vi "Baseline Thresholding.vi"(4 "Baseline Threshold Parameters":T1={"Current"=[20, 20, 20, 20, 20], "Pulse Duration"=[500, 500, 500, 500]}, 5 "Stimulator":T5={"Stim Open Data"={"Name"="", "Mode"=enum."LIVE", "Visa Timeout"=0}, "Stim Init Data"={"Frequency"=0.0, "N Factor"=0, "D/T Int"=0.0, "Active Channels"=[], "LF Channels"=[]}, "Stim Update Data"={"Pulse Mode"=[enum."Single"], "Current"=[], "Pulse Dur"=[]}, "Stim Status"={"Open"=FALSE, "On"=FALSE}}) -> (1 "Baseline Threshold Params Out":T1={"Current"=[20, 20, 20, 20, 20], "Pulse Duration"=[500, 500, 500, 500]} caption="Final Parameters", 2 "Stimulator Out":T5={"Stim Open Data"={"Name"="", "Mode"=enum."LIVE", "Visa Timeout"=0}, "Stim Init Data"={"Frequency"=0.0, "N Factor"=0, "D/T Int"=0.0, "Active Channels"=[], "LF Channels"=[]}, "Stim Update Data"={"Pulse Mode"=[enum."Single"], "Current"=[], "Pulse Dur"=[]}, "Stim Status"={"Open"=FALSE, "On"=FALSE}})   [LabVIEW 2019]
uses:
  Version 2/Data Type Defs/Stimulator.ctl
  Version 2/Data Type Defs/Stim Open Data.ctl
  Version 2/Data Type Defs/Stim Init Data.ctl
  Version 2/Data Type Defs/Stim Update Data.ctl
  Version 2/Data Type Defs/Pulse Mode (array).ctl
  Version 2/Data Type Defs/Stim Status.ctl
  Controls/Type Defs/Baseline Threshold Params.ctl
  Controls/Stim Current Array.ctl
  Controls/Pulse Duration Array.ctl
panel:
  out "Stim Open Data.Mode":enum16{"LIVE", "SIM"}(ring)
  out "Stimulator":refnum<visa-resource-name>
  out "Final Parameters":T1={"Current"=[20, 20, 20, 20, 20], "Pulse Duration"=[500, 500, 500, 500]}
  in  "Controls":T4={"Channel"=[], "PW"=340, "Current"=60} {"Current" max=126 step=2; "PW" min=20 max=500 step=5 scale=0.0..500.0}
  in  "Done":bool
  # "Gluteals"
  # "Hamstrings"
  # "Quads"
  # "TA/Dorsi"
  # "TS/Plantar"
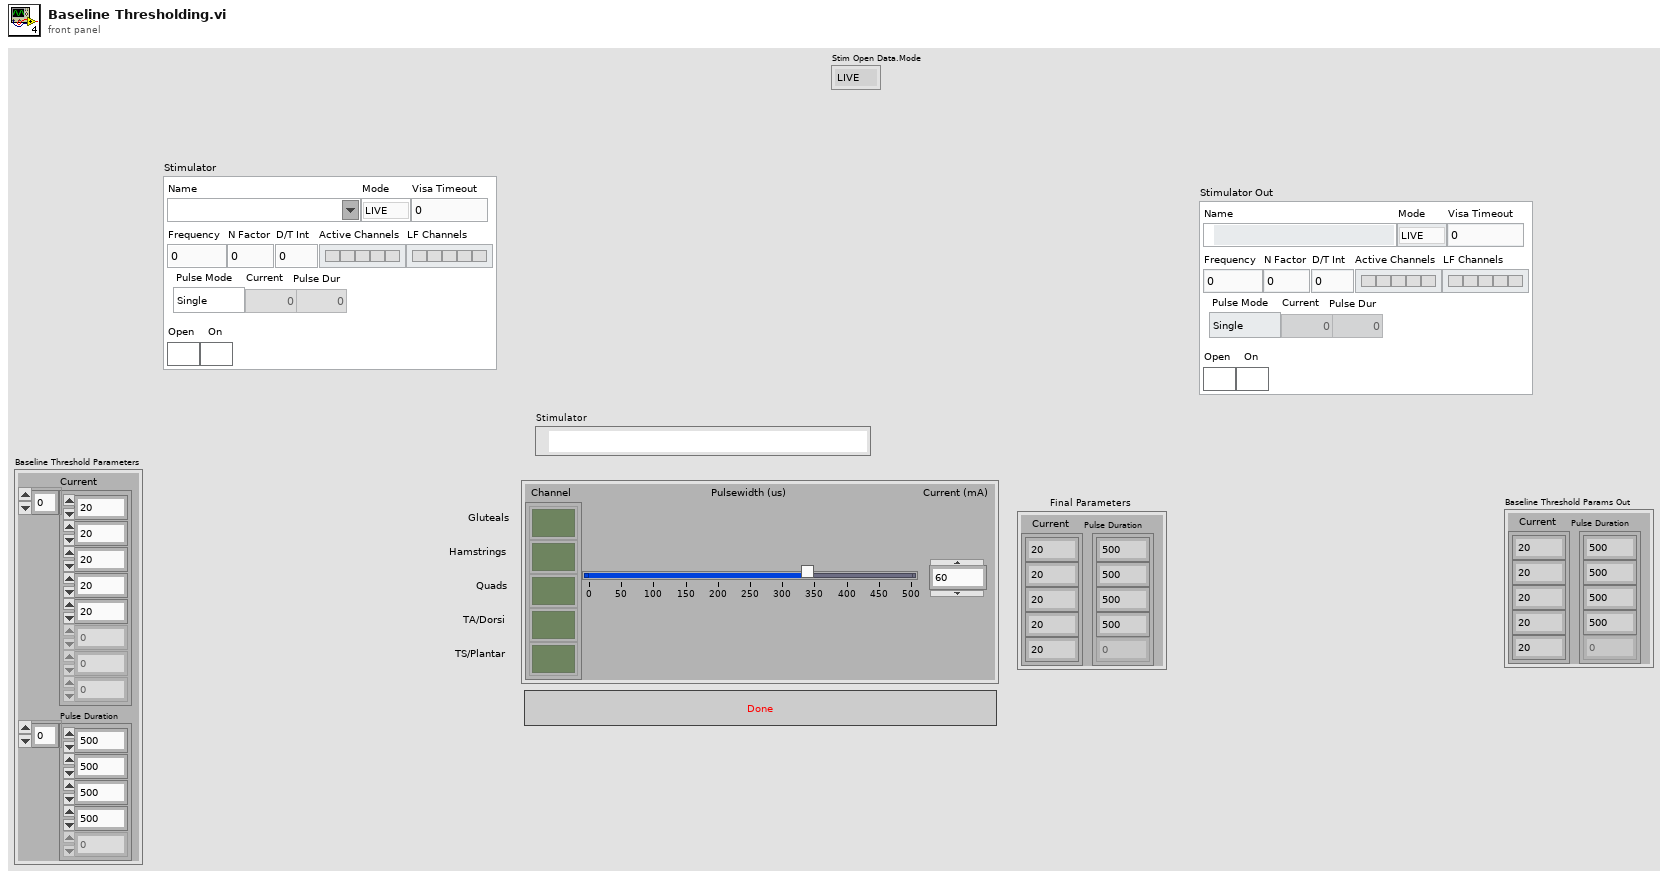
[diagram p1: front panel]
types:
  T1 = typedef "Baseline Threshold Params.ctl" = cluster{"Current":T2, "Pulse Duration":T3}
  T2 = typedef "Stim Current Array.ctl" = u8[]
  T3 = typedef "Pulse Duration Array.ctl" = u32[]
  T4 = cluster{"Channel":bool[], "PW":u16, "Current":u8}
  T5 = typedef "Stimulator.ctl" = cluster{"Stim Open Data":T6, "Stim Init Data":T7, "Stim Update Data":T8, "Stim Status":T10}
  T6 = typedef "Stim Open Data.ctl" = cluster{"Name":refnum<visa-resource-name>, "Mode":enum16{"LIVE", "SIM"}, "Visa Timeout":u32}
  T7 = typedef "Stim Init Data.ctl" = cluster{"Frequency":dbl, "N Factor":u8, "D/T Int":dbl, "Active Channels":bool[], "LF Channels":bool[]}
  T8 = typedef "Stim Update Data.ctl" = cluster{"Pulse Mode":T9, "Current":u32[], "Pulse Dur":u32[]}
  T9 = typedef "Pulse Mode (array).ctl" = enum16{"Single", "Doublet", "Triplet"}[]
  T10 = typedef "Stim Status.ctl" = cluster{"Open":bool, "On":bool}
  T11 = enum8{"Enabled", "Disabled", "Disabled and Grayed Out"}
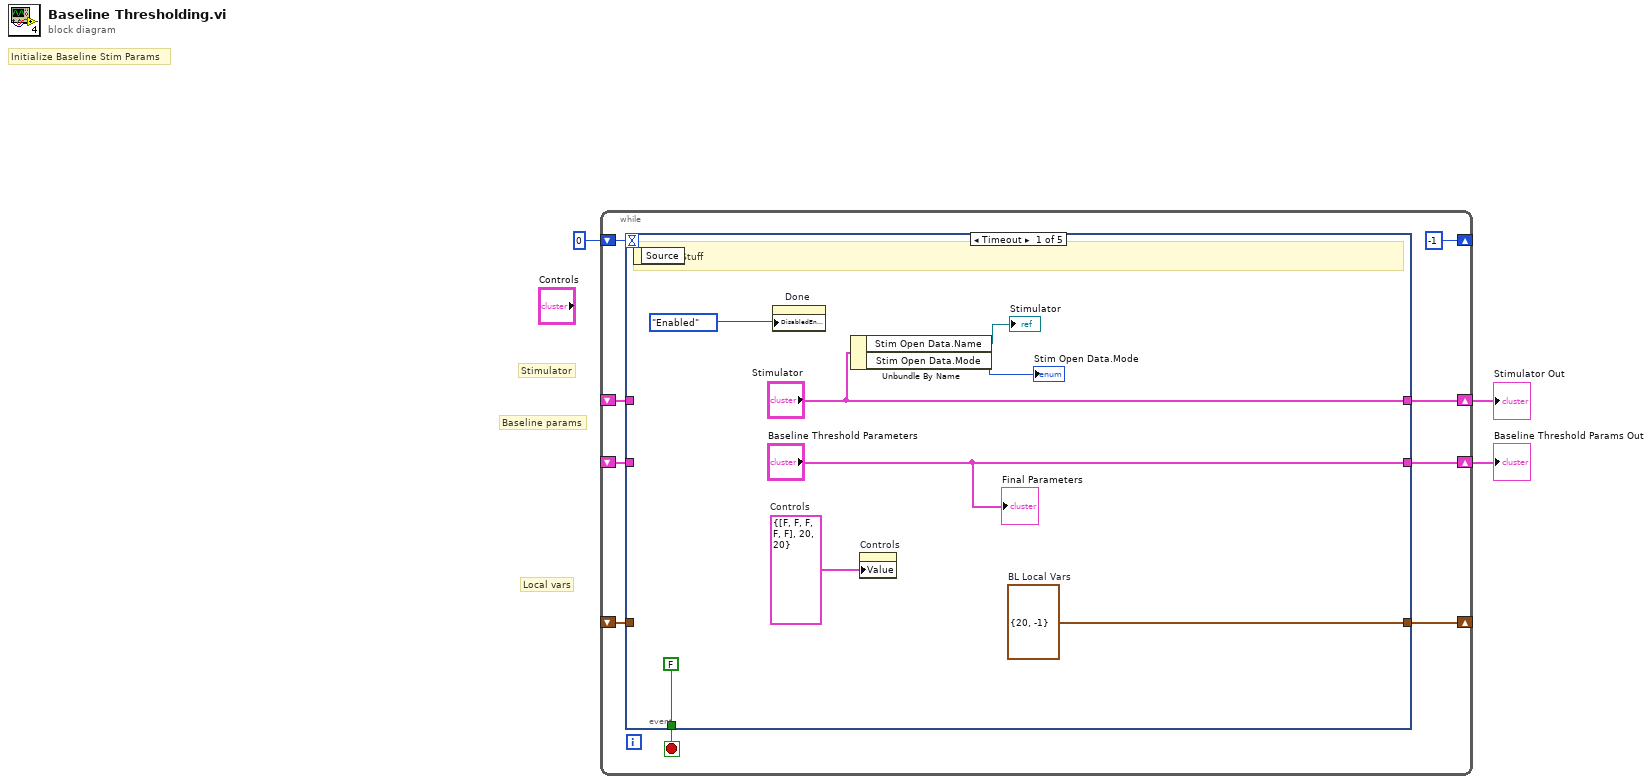
[diagram p0: block diagram]
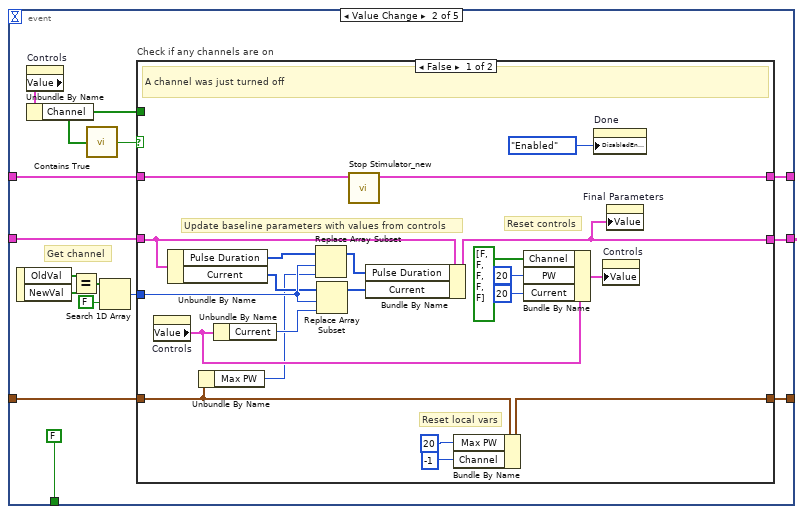
[diagram p2: hidden frame]
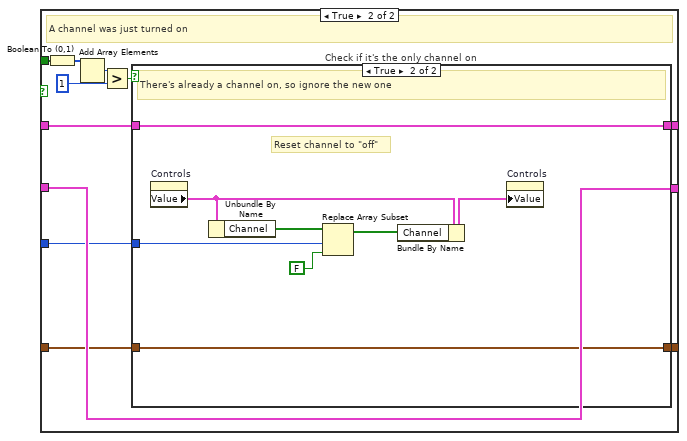
[diagram p3: hidden frame]
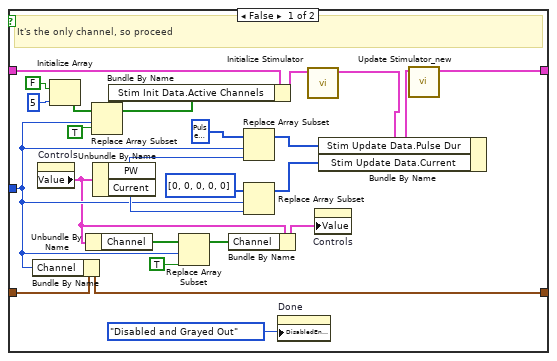
[diagram p4: hidden frame]
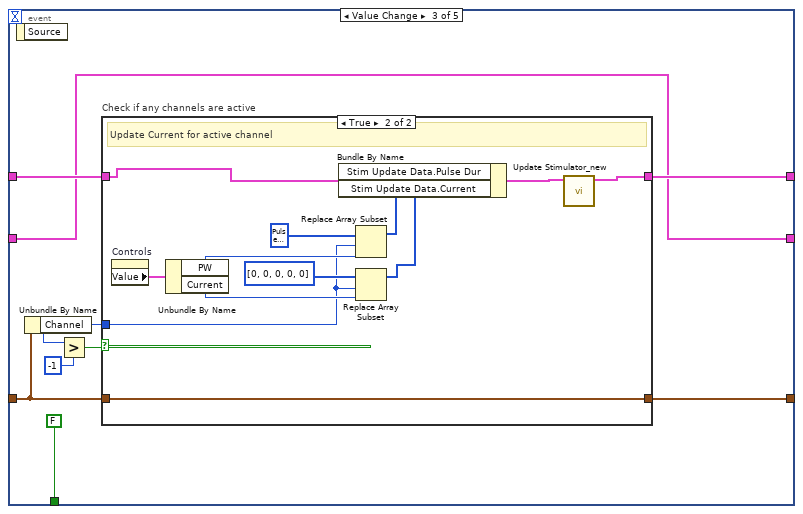
[diagram p5: hidden frame]
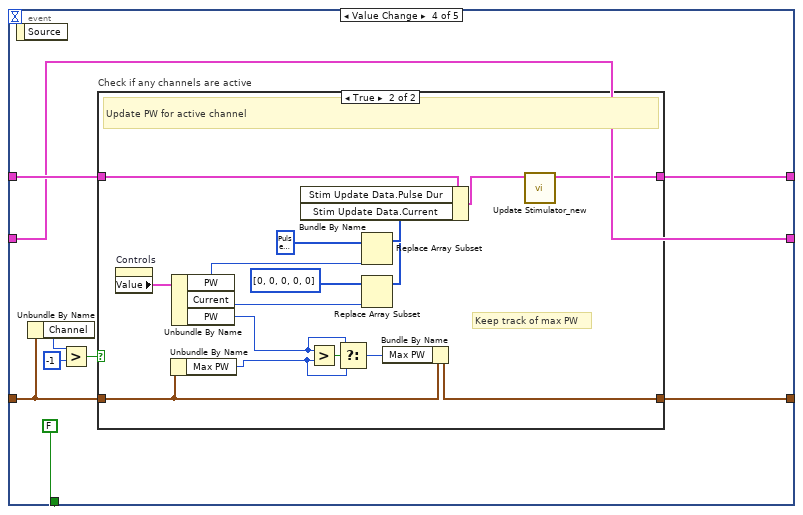
[diagram p7: hidden frame]
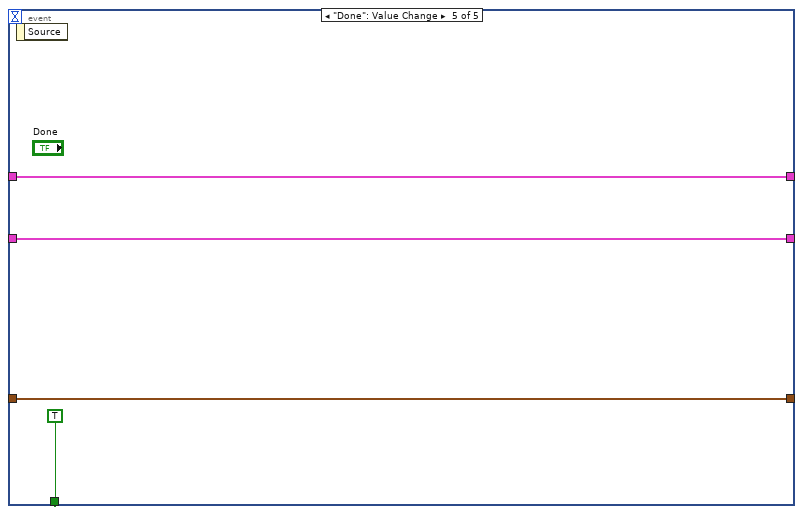
[diagram p9: hidden frame]
diagram:
  # "Local vars"
  # "Stimulator"
  # "Baseline params"
  # "Initialize Baseline Stim Params"
  n1 = while "Stim Loop" {
    shift-right: [w6] -> w1
    shift-left: _ -> [w10]
    shift-right: [w11] -> w2
    shift-left: _ -> [w9]
    shift-right: [-1] -> _
    shift-left: 0 -> [w8]
    shift-right: [w4] -> _
    shift-left: _ -> [w5]
    stop <- w12 stop-if-true
    n2 = event shown="[0] Timeout" {
      selector: _ -> [_ _ _ _ _]
      dyn-events: _ -> [_ _ _ _ _]
      timeout: w8 -> [_ _ _ _ _]
      tunnel: w9 -> [_ w34 w107 w130 w153]
      tunnel: [FALSE FALSE FALSE FALSE TRUE] -> w12
      tunnel: ["Baseline Threshold Parameters" w21 w105 w128 w152] -> w6
      tunnel: ["Stimulator" w28 w106 w129 w153] -> w11
      tunnel: w10 -> [_ w26 w105 w128 w152]
      tunnel: [w17 w24 w103 w126 w151] -> w4
      tunnel: w5 -> [_ w25 w102 w125 w151]
      event Timeout {
        w18 = T4 {"Channel"=[FALSE, FALSE, FALSE, FALSE, FALSE], "PW"=20, "Current"=20}  # Controls
        w17 = cluster{"Max PW":i32, "Channel":i32} {"Max PW"=20, "Channel"=-1}  # BL Local Vars
        # "Initialize Stuff"
        n3 = event-data() -> ()  [unwired: 1 in, 1 out]
        n4 = property on="Done" class="Bool"("DisabledEnum"=T11."Enabled" ("Disabled")) -> ()  [unwired: 2 in, 2 out]
        n5 = Unbundle By Name("Stimulator") -> ("Stim Open Data.Name"=→"Stimulator":refnum<visa-resource-name>, "Stim Open Data.Mode"=→"Stim Open Data.Mode":enum16{"LIVE", "SIM"})
        n6 = property on="Controls" class="Clust (strict)"("Value"=w18) -> ()  [unwired: 2 in, 2 out]
        "Final Parameters" <- "Baseline Threshold Parameters"
      }
      event "Controls.Channel": Value Change {
        # "Get channel"
        n7 = event-data() -> ("OldVal"=w32:bool[], "NewVal"=w31:bool[])  [unwired: 1 in]
        n8 = property on="Controls" class="Clust (strict)"() -> ("Value"=w23:T4)  [unwired: 2 in, 2 out]
        n9 = Unbundle By Name(w23) -> ("Channel"=w22:bool[])
        n10 = Equal?(x=w32, y=w31) -> (x = y?=w30:bool[])
        n11 = call "Contains True.vi"("R Channel BL"=w22) -> ("Boolean"=w35:bool)
        n12 = Search 1D Array(1D array=w30, element=FALSE) -> (index of element=w29:i32)  [unwired: 1 in]
        n13 = case "Check if any channels are on" shown="False" w35 {
          tunnel: w34 -> [w54 w64]
          tunnel: w29 -> [w55 w61]
          tunnel: [w53 w63] -> w28
          tunnel: w26 -> [w42 w62]
          tunnel: [w36 w62] -> w21
          tunnel: w25 -> [w38 w60]
          tunnel: [w39 w59] -> w24
          tunnel: w22 -> [_ w58]
          frame False {
            # "Reset local vars"
            # "Reset controls"
            # "Update baseline parameters with values from controls"
            # "A channel was just turned off"
            n14 = property on="Controls" class="Clust (strict)"() -> ("Value"=w43:T4)  [unwired: 2 in, 2 out]
            n15 = Unbundle By Name(w42) -> ("Pulse Duration"=w41:T3, "Current"=w40:T2)
            n16 = Unbundle By Name(w38) -> ("Max PW"=w37:i32)
            n17 = Unbundle By Name(w43) -> ("Current"=w46:u8)
            n18 = Replace Array Subset(array=w41, new element=w37, index=w55) -> (w45:T3)
            n19 = Replace Array Subset(array=w40, new element=w46, index=w55) -> (w44:T2)
            n20 = call "Stop Stimulator_new.vi"("Stimulator"=w54) -> ("Stimulator Out"=w53:T5)  [unwired: 3 in, 3 out]
            n21 = Bundle By Name(cluster=w42, "Pulse Duration"=w45, "Current"=w44) -> (w36:T1)
            n22 = Bundle By Name(cluster=w38, "Max PW"=20, "Channel"=-1) -> (w39:cluster{"Max PW":i32, "Channel":i32})
            n23 = Bundle By Name(cluster=w43, "Channel"=bool[] [FALSE, FALSE, FALSE, FALSE, FALSE] ("Channel Indicator"), "PW"=20 ("Pulse duration"), "Current"=20) -> (w50:T4)
            n24 = property on="Done" class="Bool"("DisabledEnum"=T11."Enabled" ("Disabled")) -> ()  [unwired: 2 in, 2 out]
            n25 = property on="Controls" class="Clust (strict)"("Value"=w50) -> ()  [unwired: 2 in, 2 out]
            n26 = property on="Final Parameters" class="Clust (strict)"("Value"=w36) -> ()  [unwired: 2 in, 2 out]
          }
          frame True {
            # "A channel was just turned on"
            n27 = Boolean To (0,1)(Boolean=w58) -> (0, 1=w57:i16[])
            n28 = Add Array Elements(numeric array=w57) -> (sum=w67:i16)
            n29 = Greater?(x=w67, y=i16 1) -> (0:w65:bool)
            n30 = case "Check if it's the only channel on" shown="True" w65 {
              tunnel: w64 -> [w89 w99]
              tunnel: [w92 w99] -> w63
              tunnel: w61 -> [w76 w97]
              tunnel: [w70 w93] -> w59
              tunnel: w60 -> [w71 w93]
              frame False {
                # "It's the only channel, so proceed"
                n31 = Bundle By Name(cluster=w71, "Channel"=w76) -> (w70:cluster{"Max PW":i32, "Channel":i32})
                n32 = property on="Controls" class="Clust (strict)"() -> ("Value"=w74:T4)  [unwired: 2 in, 2 out]
                n33 = Initialize Array(FALSE ("new element/subarray"), 5 ("dimension size")) -> (w86:bool[])
                n34 = Unbundle By Name(w74) -> ("Channel"=w78:bool[])
                n35 = Replace Array Subset(array=w86, new element=TRUE ("new element/subarray"), index=w76) -> (w87:bool[])
                n36 = Unbundle By Name(w74) -> ("PW"=w79:u16, "Current"=w80:u8)
                n37 = Bundle By Name(cluster=w89, "Stim Init Data.Active Channels"=w87) -> (w68:T5)
                n38 = Replace Array Subset(array=w78, new element=TRUE ("new element/subarray"), index=w76) -> (w75:bool[])
                n39 = Bundle By Name(cluster=w74, "Channel"=w75) -> (w73:T4)
                n40 = Replace Array Subset(array=T3 [0, 0, 0, 0, 0] ("Pulse Duration"), new element=w79, index=w76) -> (w91:T3)
                n41 = Replace Array Subset(array=T2 [0, 0, 0, 0, 0] ("Current"), new element=w80, index=w76) -> (w90:T2)
                n42 = property on="Done" class="Bool"("DisabledEnum"=T11."Disabled and Grayed Out" ("Disabled")) -> ()  [unwired: 2 in, 2 out]
                n43 = call "Initialize Stimulator.vi"("Stimulator"=w68) -> ("Stimulator"=w69:T5)  [unwired: 3 in, 3 out]
                n44 = property on="Controls" class="Clust (strict)"("Value"=w73) -> ()  [unwired: 2 in, 2 out]
                n45 = Bundle By Name(cluster=w69, "Stim Update Data.Pulse Dur"=w91, "Stim Update Data.Current"=w90) -> (w83:T5)
                n46 = call "Update Stimulator_new.vi"("Stimulator"=w83) -> ("Stimulator"=w92:T5)  [unwired: 3 in, 3 out]
              }
              frame True {
                # "Reset channel to \"off\""
                # "There's already a channel on, so ignore the new one"
                n47 = property on="Controls" class="Clust (strict)"() -> ("Value"=w96:T4)  [unwired: 2 in, 2 out]
                n48 = Unbundle By Name(w96) -> ("Channel"=w98:bool[])
                n49 = Replace Array Subset(array=w98, new element=FALSE ("new element/subarray"), index=w97) -> (w94:bool[])
                n50 = Bundle By Name(cluster=w96, "Channel"=w94) -> (w95:T4)
                n51 = property on="Controls" class="Clust (strict)"("Value"=w95) -> ()  [unwired: 2 in, 2 out]
              }
            }
          }
        }
      }
      event "Controls.Current": Value Change {
        n52 = event-data() -> ()  [unwired: 1 in, 1 out]
        n53 = Unbundle By Name(w102) -> ("Channel"=w101:i32)
        n54 = Greater?(x=w101, y=-1) -> (0:w108:bool)
        n55 = case "Check if any channels are active" shown="True" w108 {
          tunnel: w107 -> [w111 w113]
          tunnel: [w111 w123] -> w106
          tunnel: w102 -> [w110 w115]
          tunnel: [w110 w115] -> w103
          tunnel: w101 -> [_ w114]
          frame False {
            # "No channels active, do nothing"
          }
          frame True {
            # "Update Current for active channel"
            n56 = property on="Controls" class="Clust (strict)"() -> ("Value"=w116:T4)  [unwired: 2 in, 2 out]
            n57 = Unbundle By Name(w116) -> ("PW"=w117:u16, "Current"=w118:u8)
            n58 = Replace Array Subset(array=T3 [0, 0, 0, 0, 0] ("Pulse Duration"), new element=w117, index=w114) -> (w121:T3)
            n59 = Replace Array Subset(array=T2 [0, 0, 0, 0, 0] ("Current"), new element=w118, index=w114) -> (w122:T2)
            n60 = Bundle By Name(cluster=w113, "Stim Update Data.Pulse Dur"=w121, "Stim Update Data.Current"=w122) -> (w112:T5)
            n61 = call "Update Stimulator_new.vi"("Stimulator"=w112) -> ("Stimulator"=w123:T5)  [unwired: 3 in, 3 out]
          }
        }
      }
      event "Controls.PW": Value Change {
        n62 = event-data() -> ()  [unwired: 1 in, 1 out]
        n63 = Unbundle By Name(w125) -> ("Channel"=w124:i32)
        n64 = Greater?(x=w124, y=-1) -> (0:w131:bool)
        n65 = case "Check if any channels are active" shown="True" w131 {
          tunnel: w130 -> [w134 w136]
          tunnel: [w134 w149] -> w129
          tunnel: w125 -> [w133 w139]
          tunnel: [w133 w138] -> w126
          frame False {
            # "No channels active, do nothing"
          }
          frame True {
            # "Keep track of max PW"
            # "Update PW for active channel"
            n66 = property on="Controls" class="Clust (strict)"() -> ("Value"=w143:T4)  [unwired: 2 in, 2 out]
            n67 = Unbundle By Name(w139) -> ("Max PW"=w137:i32)
            n68 = Unbundle By Name(w143) -> ("PW"=w144:u16, "Current"=w145:u8, "PW"=w140:u16)
            n69 = Greater?(x=w140, y=w137) -> (0:w150:bool)
            n70 = Select(t=w140, s=w150, f=w137) -> (s? t:f=w148:i32)
            n71 = Replace Array Subset(array=T3 [0, 0, 0, 0, 0] ("Pulse Duration"), new element=w144) -> (w142:T3)  [unwired: 1 in]
            n72 = Replace Array Subset(array=T2 [0, 0, 0, 0, 0] ("Current"), new element=w145) -> (w141:T2)  [unwired: 1 in]
            n73 = Bundle By Name(cluster=w136, "Stim Update Data.Pulse Dur"=w142, "Stim Update Data.Current"=w141) -> (w135:T5)
            n74 = Bundle By Name(cluster=w139, "Max PW"=w148) -> (w138:cluster{"Max PW":i32, "Channel":i32})
            n75 = call "Update Stimulator_new.vi"("Stimulator"=w135) -> ("Stimulator"=w149:T5)  [unwired: 3 in, 3 out]
          }
        }
      }
      event "Done": Value Change {
        n76 = event-data() -> ()  [unwired: 1 in, 1 out]
      }
    }
  }
  "Stimulator Out" <- w2
  "Baseline Threshold Params Out" <- w1
